vi "UDP Data Link - RTMs - Add Channels Updated.vi"(8 "error in (no error)":errorcluster, 11 "Node Ptr":u64 format="%.0x") -> (0 "error out":errorcluster)   [LabVIEW 2012, in "UDP Data Link System Explorer.lvlib"]
uses:
  UDP Data Link System Explorer.lvlib
  <vilib>/NI Veristand/Custom Device API/Custom Device Item Ref.ctl
  <vilib>/NI Veristand/Custom Device API/Custom Device Channel Type.ctl
  Shared/UDP Data Link Global.vi
  <vilib>/NI Veristand/Custom Device API/Get Item Property (String Array).vi
  <vilib>/NI Veristand/Custom Device API/Set Item Property (String Array).vi
  <vilib>/NI Veristand/Custom Device API/Custom Device API.lvlib
  <vilib>/NI Veristand/Custom Device Tools/Custom Device Utility Library/Custom Device Utility Library.lvlib
  Shared/UDP Data Link Shared.lvlib
panel:
  in  "Remove":bool
  in  "Selected Channels":i32[](listbox)
  in  "Add":bool
  in  "Available Channels":string[](tree)
  in  "OK":bool
  in  "Cancel":bool
  in  "Initial Selection":T1[](array[typedef]) format="%.0x"
  in  "Tag":string
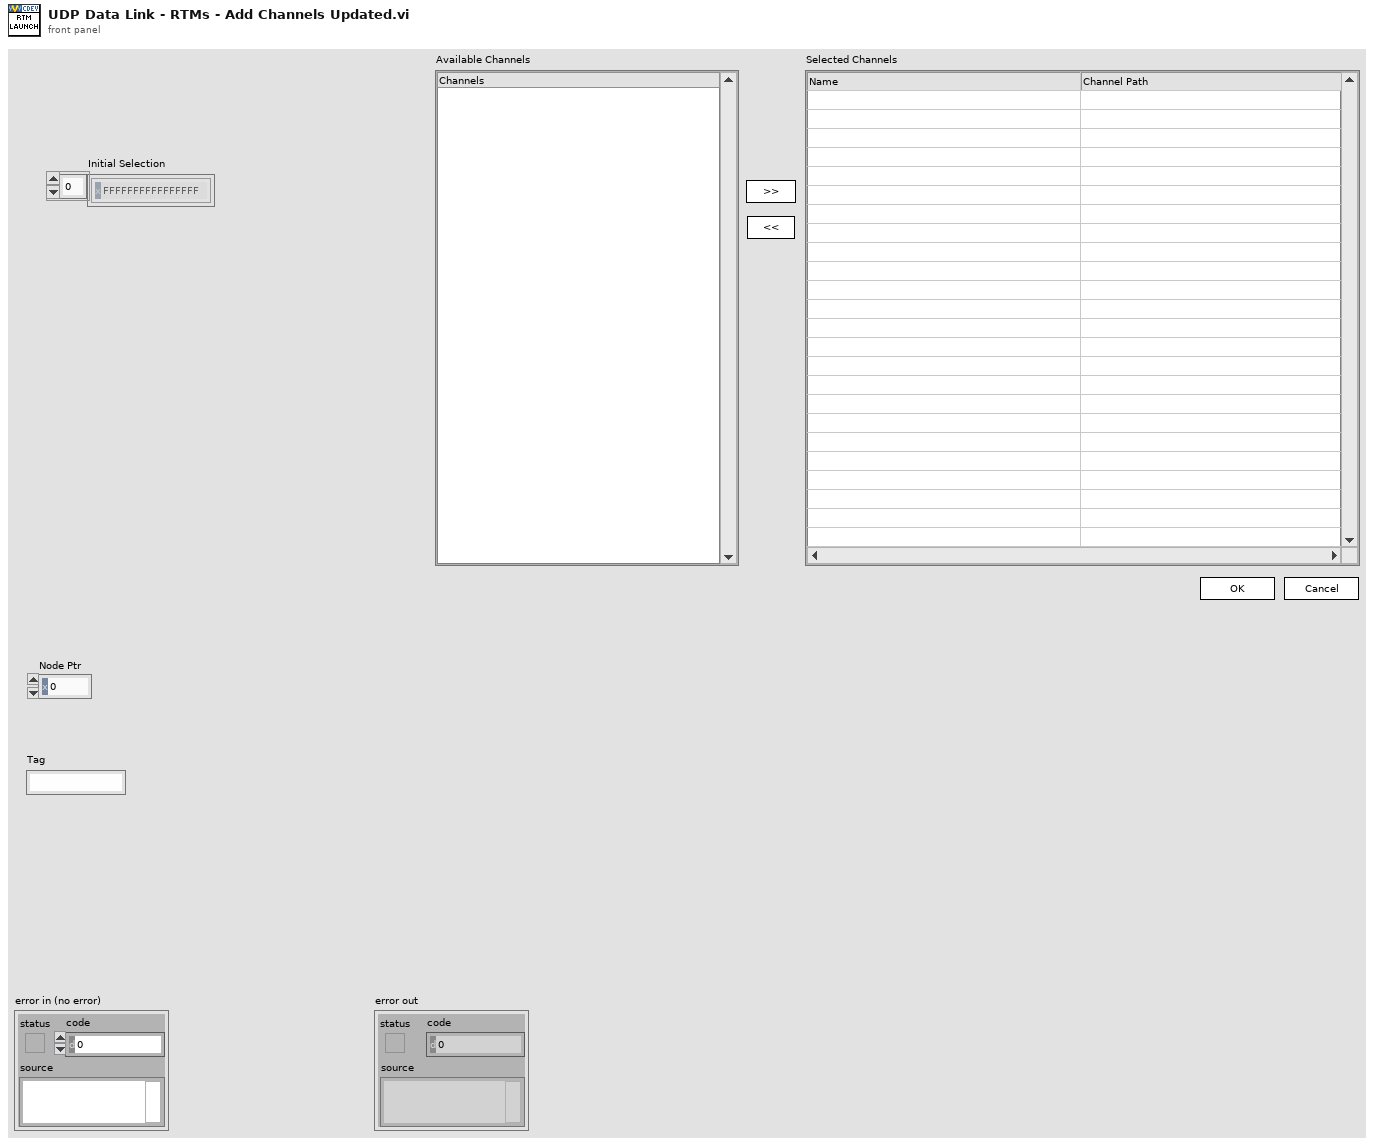
[diagram p1: front panel]
types:
  T1 = typedef "Custom Device API.lvlib/Custom Device Item Ref.ctl" = u64
  T2 = cluster{"Allow Section Selection (F)":bool, "Allow Multiple Selection (F)":bool}
  T3 = cluster{"Available Channels Label":string, "Selected Channels Label":string, "Mode":enum16{"Tx", "Rx"}}
  T4 = enum8{"Enabled", "Disabled", "Disabled and Grayed Out"}
  T5 = typedef "Custom Device API.lvlib/Custom Device Channel Type.ctl" = enum16{"Input", "Output"}
  T6 = cluster{"Tx Channel Refs":string, "Tx Channel Paths":string, "Tx Channel Names":string, "Item Ref out":T1}
  T7 = typedef "LVRowAndColumnUnsignedTypeDef.ctl" = cluster{"Row":u32, "Column":u32}
  T8 = typedef "Custom Device API.lvlib/Custom Device Item Info.ctl" = cluster{"Name":string, "Is Channel":bool, "GUID":string, "Is Waveform":bool}
  T9 = typedef "Custom Device API.lvlib/Custom Device Channel.ctl" = cluster{"Type":T5, "Units":string, "Default Value":dbl, "Faultable":bool, "Scalable":bool}
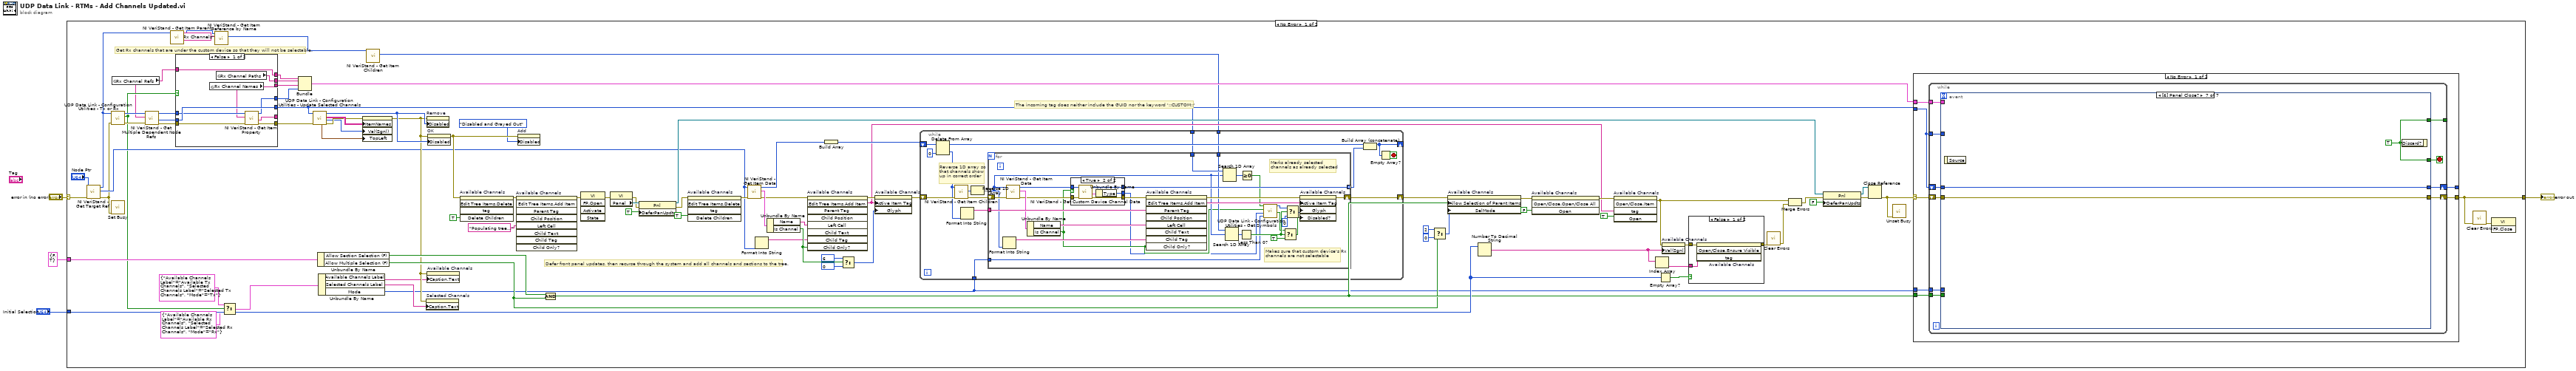
[diagram p0: block diagram]
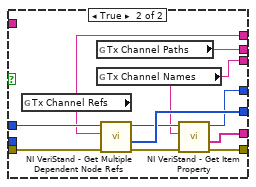
[diagram p2: hidden frame]
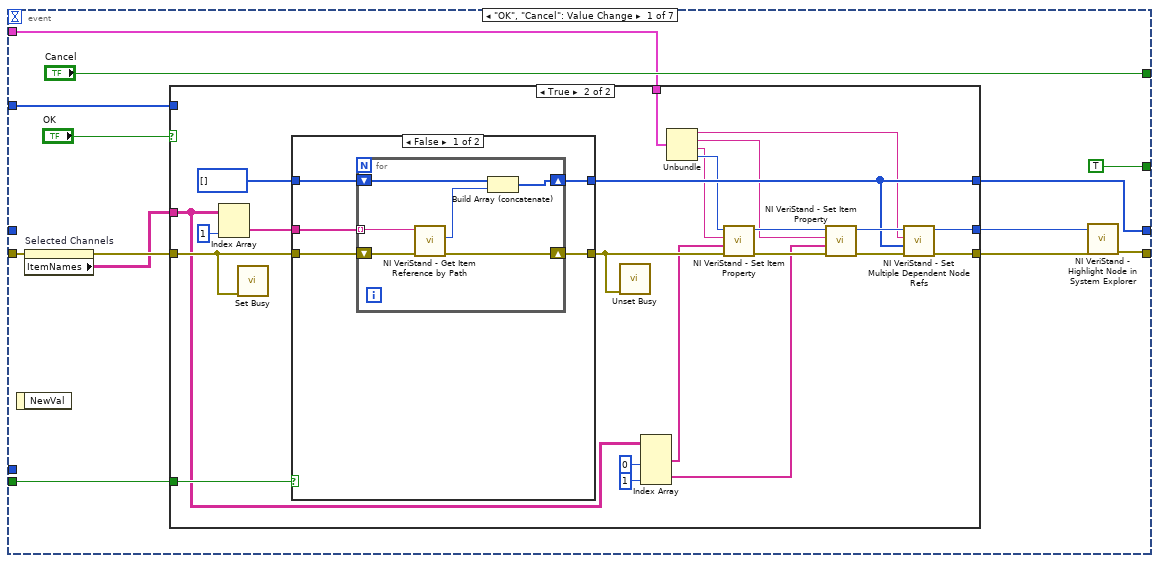
[diagram p4: hidden frame]
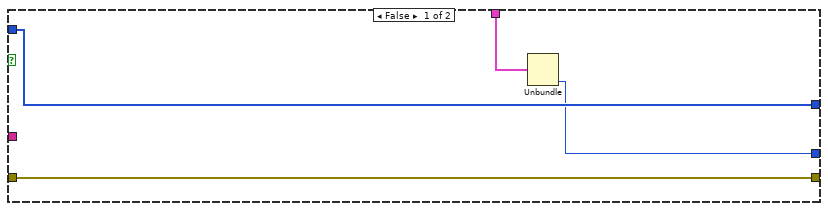
[diagram p5: hidden frame]
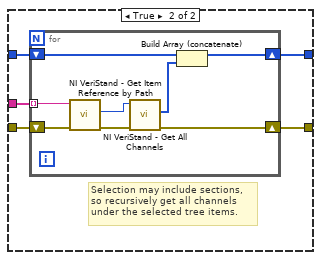
[diagram p6: hidden frame]
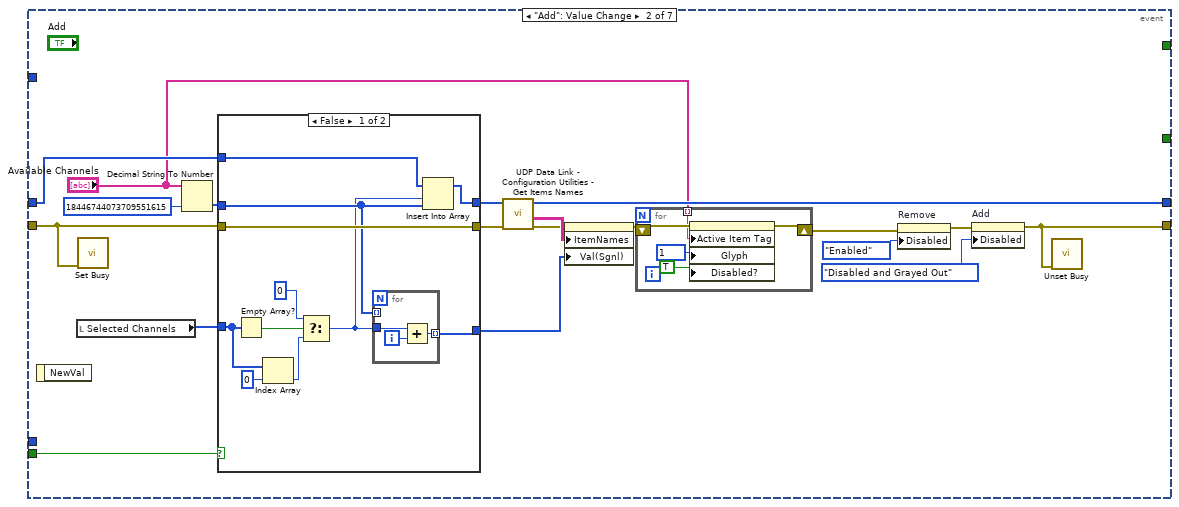
[diagram p7: hidden frame]
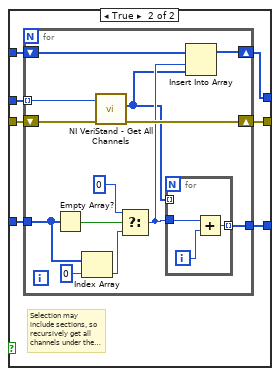
[diagram p8: hidden frame]
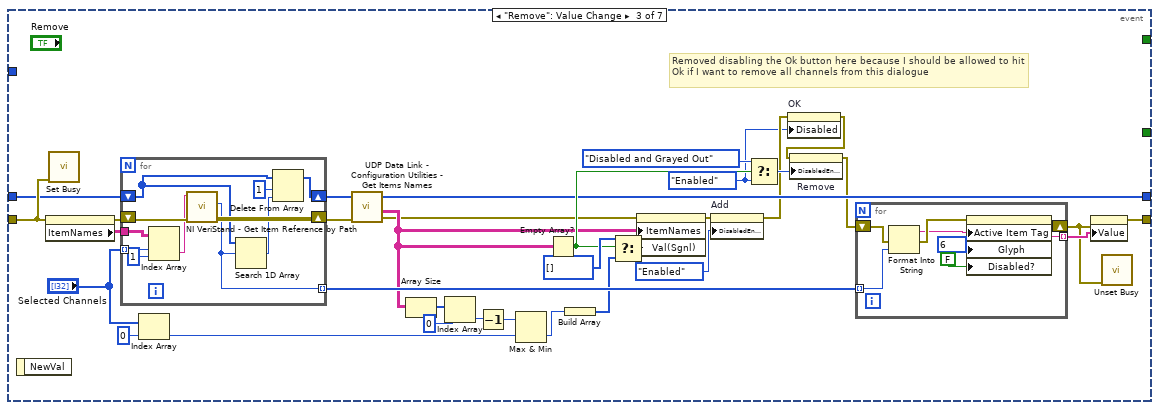
[diagram p9: hidden frame]
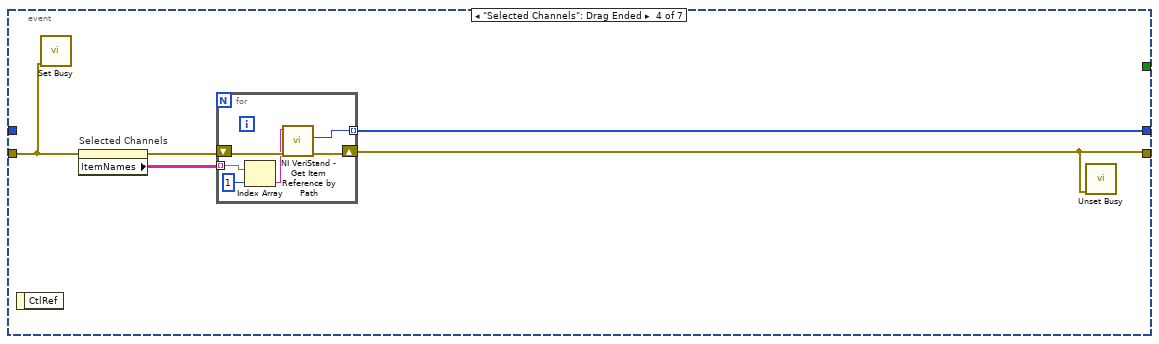
[diagram p10: hidden frame]
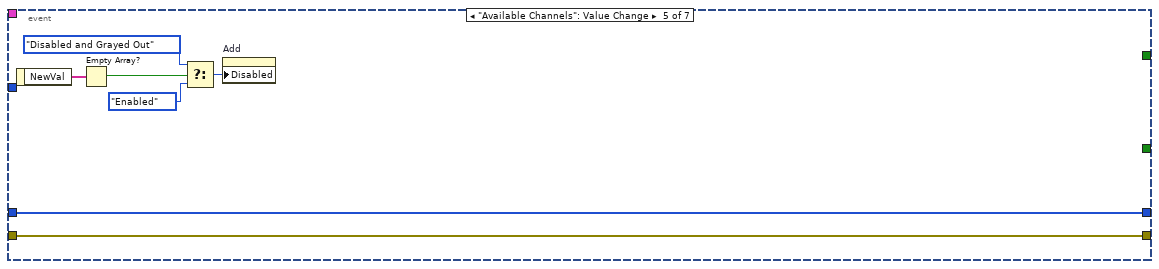
[diagram p11: hidden frame]
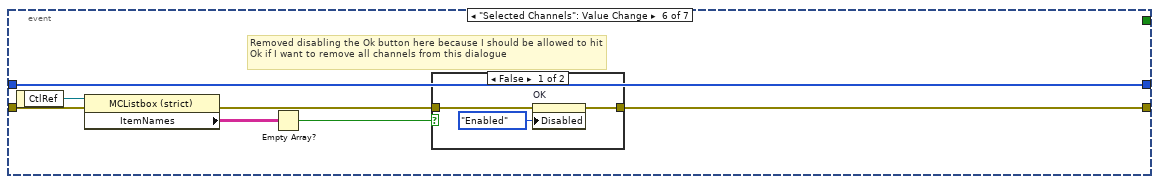
[diagram p12: hidden frame]
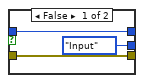
[diagram p15: hidden frame]
diagram:
  # "The incoming tag does neither include the GUID nor the keyword '::CUSTOM::'"
  n1 = case shown="No Error" "error in (no error)" {
    selector: "error in (no error)" -> [w27 w397]
    tunnel: "Initial Selection" -> [w59 _]
    tunnel: [w77 w397] -> w1
    tunnel: T2 {"Allow Section Selection (F)"=FALSE, "Allow Multiple Selection (F)"=TRUE} ("Cluster") -> [w44 _]
    frame No Error {
      # "Get Rx channels that are under the custom device so that they will not be selectable."
      # "Defer front panel updates, then recurse through the system and add all channels and sections to the tree."
      n2 = call <vilib>:"NI VeriStand - Get Target Ref.vi"("error in"=w27, "Item Ref in"="Node Ptr") -> ("error out"=w24:errorcluster, "Target Ref"=w25:T1, "Item Ref out"=w8:T1)  [unwired: 6 in, 1 out]
      n3 = call <vilib>:"Set Busy.vi"("error in (no error)"=w24) -> ()  [unwired: 3 in, 8 out]
      n4 = call "UDP Data Link - Configuration Utilities - Tx or Rx.vi"("error in (no error)"=w24, "Item Ref in"=w8) -> ("error out"=w23:errorcluster, "Tx?"=w19:bool, "Item Ref out"=w22:T1)  [unwired: 7 in]
      n5 = global read "UDP Data Link Global.vi" "Rx Channel Refs"() -> (w13:string)
      n6 = call <vilib>:"NI VeriStand - Get Multiple Dependent Node Refs.vi"("error in (no error)"=w23, "Base Property Name"=w13, "Item Ref in"=w22) -> ("error out"=w28:errorcluster, "Dependent Node Refs"=w11:T1[], "Item Ref out"=w29:T1)  [unwired: 6 in]
      n7 = call <vilib>:"NI VeriStand - Get Item Parent.vi"("Item Ref in"=w8) -> ("Parent Ref"=w6:T1)  [unwired: 7 in, 3 out]
      n8 = case shown="False" w19 {
        tunnel: w29 -> [w99 w113]
        tunnel: [w100 w112] -> w31
        tunnel: w28 -> [w96 w111]
        tunnel: [w95 w108] -> w30
        tunnel: [w94 w107] -> _
        tunnel: w11 -> [w100 _]
        tunnel: [w102 w106] -> w17
        tunnel: [w97 w105] -> w16
        tunnel: [w98 w104] -> w10
        tunnel: [w101 w103] -> w14
        tunnel: w13 -> [w101 _]
        frame False {
          n9 = global read "UDP Data Link Global.vi" "Rx Channel Names"() -> (w97:string)
          n10 = global read "UDP Data Link Global.vi" "Rx Channel Paths"() -> (w102:string)
          n11 = call-poly <vilib>:"NI VeriStand - Get Item Property.vi"("error in (no error)"=w96, "Property Name"=w97, "Item Ref in"=w99) -> ("error out"=w95:errorcluster, "Value"=w94:string[], "Item Ref out"=w98:T1)  [unwired: 1 in, 5 out]
        }
        frame True {
          n12 = global read "UDP Data Link Global.vi" "Tx Channel Refs"() -> (w103:string)
          n13 = global read "UDP Data Link Global.vi" "Tx Channel Paths"() -> (w106:string)
          n14 = global read "UDP Data Link Global.vi" "Tx Channel Names"() -> (w105:string)
          n15 = call <vilib>:"NI VeriStand - Get Multiple Dependent Node Refs.vi"("error in (no error)"=w111, "Base Property Name"=w103, "Item Ref in"=w113) -> ("error out"=w109:errorcluster, "Dependent Node Refs"=w112:T1[], "Item Ref out"=w110:T1)  [unwired: 6 in]
          n16 = call-poly <vilib>:"NI VeriStand - Get Item Property.vi"("error in (no error)"=w109, "Property Name"=w105, "Item Ref in"=w110) -> ("error out"=w108:errorcluster, "Value"=w107:string[], "Item Ref out"=w104:T1)  [unwired: 1 in, 5 out]
        }
      }
      n17 = call <vilib>:"NI VeriStand - Get Item Reference by Name.vi"("Item Name"="Rx Channels", "Parent Ref in"=w6) -> ("Item Ref"=w5:T1)  [unwired: 6 in, 3 out]
      n18 = Select(t=T3 {"Available Channels Label"="Available Tx Channels", "Selected Channels Label"="Selected Tx Channels", "Mode"=enum."Tx"} ("Parameter"), s=w19, f=T3 {"Available Channels Label"="Available Rx Channels", "Selected Channels Label"="Selected Rx Channels", "Mode"=enum."Rx"} ("Parameter")) -> (s? t:f=w18:T3)
      n19 = Bundle("Tx Channel Refs"=w14, "Tx Channel Paths"=w17, "Tx Channel Names"=w16, "Item Ref out"=w10) -> (w15:T6)  [unwired: 1 in]
      n20 = call "UDP Data Link - Configuration Utilities - Update Selected Channels.vi"("error in (no error)"=w30, "Dependent Node Refs"=w31) -> ("error out"=w40:errorcluster, "Val(Sgnl)"=w36:i32[], "Selected Channels"=w41:string[][], "Disabled Behavior"=w37:u8, "Top Left Visible Cell"=w12:T7)  [unwired: 5 in]
      n21 = Unbundle By Name(w44) -> ("Allow Section Selection (F)"=w43:bool, "Allow Multiple Selection (F)"=w42:bool)
      n22 = Unbundle By Name(w18) -> ("Available Channels Label"=w34:string, "Selected Channels Label"=w33:string, "Mode"=w32:enum16{"Tx", "Rx"})
      n23 = property on="Selected Channels" class="MCListbox (strict)"(error in=w40, "ItemNames"=w41, "Val(Sgnl)"=w36, "TopLeft"=w12) -> (error out=w35:errorcluster)  [unwired: 1 in, 1 out]
      n24 = call <vilib>:"NI VeriStand - Get Item Children.vi"("Item Ref in"=w5) -> ("Child Refs"=w9:T1[])  [unwired: 7 in, 3 out]
      n25 = property on="Selected Channels" class="MCListbox (strict)"(error in=w35, "Caption.Text"=w33) -> ()  [unwired: 1 in, 2 out]
      n26 = property on="Remove" class="Bool"(error in=w35, "Disabled"=w37) -> ()  [unwired: 1 in, 2 out]
      n27 = property on="Available Channels" class="Tree (strict)"(error in=w35, "Caption.Text"=w34) -> ()  [unwired: 1 in, 2 out]
      n28 = property on="OK" class="Bool"(error in=w35, "Disabled"=w37) -> (error out=w39:errorcluster)  [unwired: 1 in, 1 out]
      n29 = invoke on="Available Channels" class="Tree (strict)" method="Edit Tree Items.Delete"(error in=w39, "Delete Children"=TRUE ("Delete Children?")) -> (error out=w93:errorcluster)  [unwired: 3 in, 4 out]
      n30 = invoke on="Available Channels" class="Tree (strict)" method="Edit Tree Items.Add Item"(error in=w93, "Left Cell"="Populating tree..." ("Tag")) -> (error out=w90:errorcluster)  [unwired: 7 in, 8 out]
      n31 = property on="Add" class="Bool"(error in=w39, "Disabled"=T4."Disabled and Grayed Out") -> ()  [unwired: 1 in, 2 out]
      n32 = Compound Arithmetic op=AND(w43, w42) -> (w46:bool)
      n33 = invoke class="VI" method="FP.Open"(error in=w90) -> (error out=w88:errorcluster)  [unwired: 4 in, 4 out]
      n34 = property class="VI"(error in=w88) -> (error out=w86:errorcluster, "Panel"=w87:refnum<vi>)  [unwired: 1 in, 1 out]
      n35 = property class="Pnl"(reference=w87, error in=w86, "DeferPanUpdts"=TRUE ("Defer Panel Updates")) -> (reference out=w80:refnum<vi>, error out=w84:errorcluster)
      n36 = invoke on="Available Channels" class="Tree (strict)" method="Edit Tree Items.Delete"(error in=w84, "Delete Children"=TRUE ("Delete Children?")) -> (error out=w64:errorcluster)  [unwired: 3 in, 4 out]
      n37 = call <vilib>:"NI VeriStand - Get Item Data.vi"("error in (no error)"=w64, "Item Ref in"=w25) -> ("error out"=w67:errorcluster, "Item Info"=w69:T8, "Item Ref out"=w65:T1)  [unwired: 7 out]
      n38 = Format Into String(w25) -> (resulting string=w68:string)  [unwired: 3 in, 1 out]
      n39 = Unbundle By Name(w69) -> ("Name"=w70:string, "Is Channel"=w74:bool)
      n40 = invoke on="Available Channels" class="Tree (strict)" method="Edit Tree Items.Add Item"(error in=w67, "Left Cell"=w70, "Child Tag"=w68, "Child Only?"=w74) -> (error out=w71:errorcluster, "Edit Tree Items:Add Item"=w50:string)  [unwired: 5 in, 7 out]
      n41 = Build Array(w65) -> (w83:T1[])
      n42 = Select(t=6, s=w74, f=0) -> (s? t:f=w75:i32)
      n43 = property on="Available Channels" class="Tree (strict)"(error in=w71, "Active Item Tag"=w50, "Glyph"=w75) -> (error out=w66:errorcluster)  [unwired: 1 in, 1 out]
      n44 = while {
        shift-right: [w350] -> w82
        shift-left: w66 -> [w356]
        shift-right: [w355] -> _
        shift-left: w83 -> [w359]
        tunnel: w31 -> [w347]
        tunnel: w32 -> [w346]
        tunnel: w9 -> [w345]
        stop <- w354 stop-if-true
        # "Reverse 1D array so that channels show up in correct order"
        n45 = Delete From Array(array=w359, index=0) -> (deleted portion=w349:T1, array with subset deleted=w357:T1[])  [unwired: 1 in]
        n46 = call <vilib>:"NI VeriStand - Get Item Children.vi"("error in (no error)"=w356, "Item Ref in"=w349) -> ("error out"=w353:errorcluster, "Child Refs"=w352:T1[])  [unwired: 8 out]
        n47 = Format Into String(w349) -> (resulting string=w348:string)  [unwired: 3 in, 1 out]
        n48 = Reverse 1D Array(array=w352) -> (reversed array=w344:T1[])
        n49 = for {
          shift-right: [w381] -> w350
          shift-left: w353 -> [w386]
          tunnel: w344 -> [w373] mode=indexing
          tunnel: [w378] -> w351 mode=indexing
          tunnel: w348 -> [w387]
          tunnel: w347 -> [w380]
          tunnel: w346 -> [w362]
          tunnel: w345 -> [w374]
          # "Marks already selected channels as already selected"
          # "Makes sure that custom device's Rx channels are not selectable"
          n50 = Format Into String(w373) -> (resulting string=w385:string)  [unwired: 3 in, 1 out]
          n51 = call <vilib>:"NI VeriStand - Get Item Data.vi"("error in (no error)"=w386, "Item Ref in"=w373) -> ("error out"=w377:errorcluster, "Item Info"=w384:T8, "Item Ref out"=w379:T1)  [unwired: 7 out]
          n52 = Unbundle By Name(w384) -> ("Name"=w375:string, "Is Channel"=w364:bool)
          n53 = case shown="True" w364 {
            tunnel: w379 -> [w390 w396]
            tunnel: [w390 w395] -> w378
            tunnel: w377 -> [w389 w394]
            tunnel: [w389 w393] -> w376
            tunnel: [Custom_Device_Channel_Type."Input" ("Type") w391] -> w363
            frame False {
            }
            frame True {
              n54 = call <vilib>:"NI VeriStand - Get Custom Device Channel Data.vi"("error in (no error)"=w394, "Channel Ref in"=w396) -> ("error out"=w393:errorcluster, "Channel"=w392:T9, "Channel Ref out"=w395:T1)  [unwired: 4 in, 3 out]
              n55 = Unbundle By Name(w392) -> ("Type"=w391:T5)
            }
          }
          n56 = invoke on="Available Channels" class="Tree (strict)" method="Edit Tree Items.Add Item"(error in=w376, "Parent Tag"=w387, "Left Cell"=w375, "Child Tag"=w385, "Child Only?"=w364) -> (error out=w383:errorcluster, "Edit Tree Items:Add Item"=w382:string)  [unwired: 4 in, 7 out]
          n57 = Search 1D Array(1D array=w380, element=w373) -> (index of element=w366:i32)  [unwired: 1 in]
          n58 = Search 1D Array(1D array=w374, element=w373) -> (index of element=w372:i32)  [unwired: 1 in]
          n59 = Less Than 0?(x=w372) -> (x < 0?=w368:bool)
          n60 = Greater Or Equal To 0?(x=w366) -> (x >= 0?=w365:bool)
          n61 = call "UDP Data Link - Configuration Utilities - Get Symbols.vi"("Mode"=w362, "Channel Type"=w363, "Is Channel?"=w364, "Is Selected?"=w365) -> ("Disabled?"=w360:bool, "Symbole"=w361:i32)  [unwired: 6 in]
          n62 = Select(t=w360, s=w368, f=TRUE) -> (s? t:f=w371:bool)
          n63 = Select(t=w361, s=w368, f=0) -> (s? t:f=w369:i32)
          n64 = property on="Available Channels" class="Tree (strict)"(error in=w383, "Active Item Tag"=w382, "Glyph"=w369, "Disabled?"=w371) -> (error out=w381:errorcluster)  [unwired: 1 in, 1 out]
        }
        n65 = Build Array (concatenate)(w357, w351) -> (w355:T1[])
        n66 = Empty Array?(array=w355) -> (empty?=w354:bool)
      }
      n67 = Select(t=2 ("Selection Mode"), s=w42, f=0 ("Selection Mode")) -> (s? t:f=w47:i32)
      n68 = property on="Available Channels" class="Tree (strict)"(error in=w82, "Allow Selection of Parent Items"=w46, "SelMode"=w47) -> (error out=w55:errorcluster)  [unwired: 1 in, 1 out]
      n69 = Number To Decimal String(number=w59) -> (decimal integer string=w57:string[])  [unwired: 1 out]
      n70 = invoke on="Available Channels" class="Tree (strict)" method="Open/Close.Open/Close All"(error in=w55, "Open"=FALSE ("Open?")) -> (error out=w53:errorcluster)  [unwired: 2 in, 3 out]
      n71 = invoke on="Available Channels" class="Tree (strict)" method="Open/Close.Item"(error in=w53, "tag"=w50, "Open"=TRUE ("Open?")) -> (error out=w51:errorcluster)  [unwired: 2 in, 4 out]
      n72 = Index Array(array=w57) -> (element=w56:string)  [unwired: 1 in]
      n73 = Empty Array?(array=w59) -> (empty?=w58:bool)
      n74 = property on="Available Channels" class="Tree (strict)"(error in=w51, "Val(Sgnl)"=w57) -> (error out=w61:errorcluster)  [unwired: 1 in, 1 out]
      n75 = case shown="False" w58 {
        tunnel: w61 -> [w116 w117]
        tunnel: [w115 w117] -> w60
        tunnel: w56 -> [w114 _]
        frame False {
          n76 = invoke on="Available Channels" class="Tree (strict)" method="Open/Close.Ensure Visible"(error in=w116, "tag"=w114) -> (error out=w115:errorcluster)  [unwired: 2 in, 3 out]
        }
        frame True {
        }
      }
      n77 = call <vilib>:"Clear Errors.vi"("error in (no error)"=w60) -> ("error out"=w63:errorcluster)  [unwired: 6 out]
      n78 = Merge Errors(w51, w63) -> (w62:errorcluster)
      n79 = property class="Pnl"(reference=w80, error in=w62, "DeferPanUpdts"=FALSE ("Defer Panel Updates")) -> (reference out=w78:refnum<vi>, error out=w79:errorcluster)
      n80 = Close Reference(reference=w78, error in (no error)=w79) -> (error out=w45:errorcluster)
      n81 = call <vilib>:"Unset Busy.vi"("error in (no error)"=w45) -> ()  [unwired: 1 in, 10 out]
      n82 = case shown="No Error" w45 {
        selector: w45 -> [w124 w343]
        tunnel: [w123 w343] -> w77
        tunnel: [w122 w342] -> _
        tunnel: w46 -> [w121 _]
        tunnel: w31 -> [w120 w342]
        tunnel: w32 -> [w119 _]
        tunnel: w15 -> [w118 _]
        frame No Error {
          n83 = while {
            shift-right: [w133] -> w123
            shift-left: w124 -> [w134]
            tunnel: [w132] -> _
            tunnel: w121 -> [w130]
            shift-right: [w127] -> w122
            shift-left: w120 -> [w129]
            tunnel: w120 -> [w128]
            tunnel: w119 -> [w126]
            tunnel: w118 -> [w125]
            stop <- w131 stop-if-true
            n84 = event shown="[6] Panel Close?" {
              selector: _ -> [_ _ _ _ _ _ _]
              dyn-events: _ -> [_ _ _ _ _ _ _]
              timeout: _ -> [_ _ _ _ _ _ _]
              tunnel: w134 -> [w143 w215 w291 w314 w327 w332 w341]
              tunnel: [w139 w199 w264 w311 w327 w329 w341] -> w133
              tunnel: ["Cancel" _ _ _ _ _ w340] -> w132
              tunnel: [TRUE ("Discard?") _ _ _ _ _ w340] -> w131
              tunnel: [w135 w211 w270 w310 w324 w334 w339] -> w127
              tunnel: w130 -> [w145 w214 _ _ _ _ _]
              tunnel: w129 -> [_ w213 w288 _ w324 w334 w339]
              tunnel: w128 -> [w141 _ _ _ _ _ _]
              tunnel: w126 -> [_ _ _ _ _ _ _]
              tunnel: w125 -> [w138 _ _ _ _ _ _]
              event "OK", "Cancel": Value Change {
                n85 = event-data() -> ()  [unwired: 2 out]
                n86 = property on="Selected Channels" class="MCListbox (strict)"(error in=w143) -> (error out=w142:errorcluster, "ItemNames"=w140:string[][])  [unwired: 1 in, 1 out]
                n87 = case shown="True" "OK" {
                  tunnel: w140 -> [_ w163]
                  tunnel: w145 -> [_ w174]
                  tunnel: w142 -> [w151 w172]
                  tunnel: [w150 w159] -> w135
                  tunnel: [w151 w161] -> w136
                  tunnel: w141 -> [w150 _]
                  tunnel: w138 -> [w149 w160]
                  tunnel: [w148 w152] -> w137
                  frame False {
                    n88 = Unbundle(w149) -> ("Item Ref out"=w148:T1)  [unwired: 3 out]
                  }
                  frame True {
                    n89 = Index Array(array=w163, index (col)=1 ("disabled index (col)")) -> (element=w170:string[])  [unwired: 1 in]
                    n90 = call <vilib>:"Set Busy.vi"("error in (no error)"=w172) -> ()  [unwired: 3 in, 8 out]
                    n91 = case shown="False" w174 {
                      tunnel: w172 -> [w179 w190]
                      tunnel: [w175 w188] -> w159
                      tunnel: [w178 w187] -> w162
                      tunnel: T1[] [] ("Channel Refs") -> [w176 w189]
                      tunnel: w170 -> [w177 w186]
                      frame False {
                        n92 = for {
                          tunnel: w177 -> [w183] mode=indexing
                          shift-right: [w180] -> w175
                          shift-left: w176 -> [w181]
                          shift-right: [w184] -> w178
                          shift-left: w179 -> [w185]
                          n93 = call <vilib>:"NI VeriStand - Get Item Reference by Path.vi"("error in (no error)"=w185, "Item Path in"=w183) -> ("error out"=w184:errorcluster, "Item Ref"=w182:T1)  [unwired: 6 in, 2 out]
                          n94 = Build Array (concatenate)(w181, w182) -> (w180:T1[])
                        }
                      }
                      frame True {
                        # "Selection may include sections, so recursively get all channels under the selected tree items."
                        n95 = for {
                          shift-right: [w196] -> w188
                          shift-left: w189 -> [w197]
                          shift-right: [w198] -> w187
                          shift-left: w190 -> [w193]
                          tunnel: w186 -> [w194] mode=indexing
                          n96 = call <vilib>:"NI VeriStand - Get Item Reference by Path.vi"("error in (no error)"=w193, "Item Path in"=w194) -> ("error out"=w192:errorcluster, "Item Ref"=w191:T1)  [unwired: 6 in, 2 out]
                          n97 = call <vilib>:"NI VeriStand - Get All Channels.vi"("error in"=w192, "Section Ref in"=w191) -> ("error out"=w198:errorcluster, "Channel Refs"=w195:T1[])  [unwired: 8 out]
                          n98 = Build Array (concatenate)(w197, w195) -> (w196:T1[])
                        }
                      }
                    }
                    n99 = call <vilib>:"Unset Busy.vi"("error in (no error)"=w162) -> ()  [unwired: 1 in, 10 out]
                    n100 = Index Array(array=w163, index (col) #1=0 ("disabled index (col)"), index (col) #2=1 ("index (col)")) -> (element #1=w156:string[], element #2=w154:string[])  [unwired: 2 in]
                    n101 = Unbundle(w160) -> ("Tx Channel Refs"=w153:string, "Tx Channel Paths"=w155:string, "Tx Channel Names"=w157:string, "Item Ref out"=w158:T1)
                    n102 = call-poly <vilib>:"NI VeriStand - Set Item Property.vi"("error in (no error)"=w162, "Value"=w156, "Property Name"=w157, "Item Ref in"=w158) -> ("error out"=w164:errorcluster, "Item Ref out"=w165:T1)  [unwired: 5 in, 1 out]
                    n103 = call-poly <vilib>:"NI VeriStand - Set Item Property.vi"("error in (no error)"=w164, "Value"=w154, "Property Name"=w155, "Item Ref in"=w165) -> ("error out"=w168:errorcluster, "Item Ref out"=w169:T1)  [unwired: 5 in, 1 out]
                    n104 = call <vilib>:"NI VeriStand - Set Multiple Dependent Node Refs.vi"("error in (no error)"=w168, "Dependent Node Refs"=w159, "Base Property Name"=w153, "Item Ref in"=w169) -> ("error out"=w161:errorcluster, "Item Ref out"=w152:T1)  [unwired: 6 in]
                  }
                }
                n105 = call <vilib>:"NI VeriStand - Highlight Node in System Explorer.vi"("error in (no error)"=w136, "Item Ref in"=w137) -> ("error out"=w139:errorcluster)  [unwired: 8 in, 1 out]
              }
              event "Add": Value Change {
                n106 = event-data() -> ()  [unwired: 2 out]
                n107 = local read "Selected Channels"() -> (w203:i32[])
                n108 = call <vilib>:"Set Busy.vi"("error in (no error)"=w215) -> ()  [unwired: 3 in, 8 out]
                n109 = Decimal String To Number(string="Available Channels", default (0L)=T1 18446744073709551615 ("Device Item Ref")) -> (number=w217:u64[])  [unwired: 2 out]
                n110 = case shown="False" w214 {
                  tunnel: w215 -> [w233 w243]
                  tunnel: [w230 w242] -> w212
                  tunnel: w217 -> [w225 w241]
                  tunnel: [w233 w240] -> w210
                  tunnel: w213 -> [w231 w239]
                  tunnel: w203 -> [w229 w238]
                  tunnel: [w223 w237] -> w202
                  frame False {
                    n111 = Empty Array?(array=w229) -> (empty?=w232:bool)
                    n112 = Index Array(array=w229, index=0) -> (element=w227:i32)
                    n113 = Select(t=0, s=w232, f=w227) -> (s? t:f=w224:i32)
                    n114 = for {
                      tunnel: w225 -> [_] mode=indexing
                      tunnel: w224 -> [w236]
                      tunnel: [w234] -> w223 mode=indexing
                      i -> [w235]
                      n115 = Add(x=w236, y=w235) -> (x+y=w234:i32)
                    }
                    n116 = Insert Into Array(array=w231, index=w224, new element=w225) -> (w230:T1[])
                  }
                  frame True {
                    # "Selection may include sections, so recursively get all channels under the selected tree items."
                    n117 = for {
                      shift-right: [w248] -> w242
                      shift-left: w239 -> [w247]
                      shift-right: [w255] -> w240
                      shift-left: w243 -> [w256]
                      tunnel: w241 -> [w254] mode=indexing
                      tunnel: w238 -> [w249]
                      tunnel: [w246] -> w237
                      n118 = Empty Array?(array=w249) -> (empty?=w250:bool)
                      n119 = Index Array(array=w249, index=0) -> (element=w252:i32)
                      n120 = call <vilib>:"NI VeriStand - Get All Channels.vi"("error in"=w256, "Section Ref in"=w254) -> ("error out"=w255:errorcluster, "Channel Refs"=w244:T1[])  [unwired: 8 out]
                      n121 = Select(t=0, s=w250, f=w252) -> (s? t:f=w245:i32)
                      n122 = for {
                        tunnel: w245 -> [w259]
                        tunnel: [w257] -> w246 mode=indexing
                        tunnel: w244 -> [_] mode=indexing
                        i -> [w258]
                        n123 = Add(x=w259, y=w258) -> (x+y=w257:i32)
                      }
                      n124 = Insert Into Array(array=w247, index=w245, new element=w244) -> (w248:T1[])
                    }
                  }
                }
                n125 = call "UDP Data Link - Configuration Utilities - Get Items Names.vi"("error IO 2"=w210, "TCP Channel Refs In"=w212) -> ("error IO"=w205:errorcluster, "Items Names"=w206:string[][], "TCP Channel Refs Out"=w211:T1[])  [unwired: 7 in]
                n126 = property on="Selected Channels" class="MCListbox (strict)"(error in=w205, "ItemNames"=w206, "Val(Sgnl)"=w202) -> (error out=w209:errorcluster)  [unwired: 1 in, 1 out]
                n127 = for {
                  shift-right: [w221] -> w201
                  shift-left: w209 -> [w222]
                  tunnel: "Available Channels" -> [w219] mode=indexing
                  n128 = property on="Available Channels" class="Tree (strict)"(error in=w222, "Active Item Tag"=w219, "Glyph"=1, "Disabled?"=TRUE ("Active Item:Disabled?")) -> (error out=w221:errorcluster)  [unwired: 1 in, 1 out]
                }
                n129 = property on="Remove" class="Bool"(error in=w201, "Disabled"=T4."Enabled") -> (error out=w200:errorcluster)  [unwired: 1 in, 1 out]
                n130 = property on="Add" class="Bool"(error in=w200, "Disabled"=T4."Disabled and Grayed Out") -> (error out=w199:errorcluster)  [unwired: 1 in, 1 out]
                n131 = call <vilib>:"Unset Busy.vi"("error in (no error)"=w199) -> ()  [unwired: 1 in, 10 out]
              }
              event "Remove": Value Change {
                w261 = T4."Enabled" ("Disabled")
                # "Removed disabling the Ok button here because I should be allowed to hit Ok if I want to remove all channels from this dialogue"
                n132 = event-data() -> ()  [unwired: 2 out]
                n133 = property on="Selected Channels" class="MCListbox (strict)"(error in=w291) -> (error out=w290:errorcluster, "ItemNames"=w289:string[][])  [unwired: 1 in, 1 out]
                n134 = call <vilib>:"Set Busy.vi"("error in (no error)"=w291) -> ()  [unwired: 3 in, 8 out]
                n135 = for {
                  tunnel: w289 -> [w300]
                  tunnel: "Selected Channels" -> [w301] mode=indexing
                  shift-right: [w299] -> w272
                  shift-left: w290 -> [w302]
                  shift-right: [w297] -> w269
                  shift-left: w288 -> [w298]
                  tunnel: [w294] -> w287 mode=indexing
                  n136 = Index Array(array=w300, index (row)=w301, index (col)=1 ("disabled index (col)")) -> (element=w292:string)
                  n137 = call <vilib>:"NI VeriStand - Get Item Reference by Path.vi"("error in (no error)"=w302, "Item Path in"=w292) -> ("error out"=w299:errorcluster, "Item Ref"=w294:T1)  [unwired: 6 in, 2 out]
                  n138 = Search 1D Array(1D array=w298, element=w294) -> (index of element=w295:i32)  [unwired: 1 in]
                  n139 = Delete From Array(array=w298, length=1, index=w295) -> (array with subset deleted=w297:T1[])  [unwired: 1 out]
                }
                n140 = Index Array(array="Selected Channels", index=0) -> (element=w275:i32)
                n141 = call "UDP Data Link - Configuration Utilities - Get Items Names.vi"("error IO 2"=w272, "TCP Channel Refs In"=w269) -> ("error IO"=w268:errorcluster, "Items Names"=w271:string[][], "TCP Channel Refs Out"=w270:T1[])  [unwired: 7 in]
                n142 = Array Size(array=w271) -> (size(s)=w279:i32[])
                n143 = Index Array(array=w279, index=0) -> (element=w277:i32)
                n144 = Decrement(x=w277) -> (x-1=w276:i32)
                n145 = Max & Min(x=w276, y=w275) -> (min(x,y)=w274:i32)  [unwired: 1 out]
                n146 = Empty Array?(array=w271) -> (empty?=w284:bool)
                n147 = Build Array(w274) -> (w281:i32[])
                n148 = Select(t=i32[] [] ("Selected TCP Channels"), s=w284, f=w281) -> (s? t:f=w285:i32[])
                n149 = property on="Selected Channels" class="MCListbox (strict)"(error in=w268, "ItemNames"=w271, "Val(Sgnl)"=w285) -> ()  [unwired: 1 in, 2 out]
                n150 = property on="Add" class="Bool"(error in=w268, "DisabledEnum"=T4."Enabled" ("Disabled")) -> (error out=w267:errorcluster)  [unwired: 1 in, 1 out]
                n151 = Select(t=T4."Disabled and Grayed Out" ("Disabled"), s=w284, f=w261) -> (s? t:f=w283:T4)
                n152 = property on="OK" class="Bool"(error in=w267, "Disabled"=w261) -> (error out=w266:errorcluster)  [unwired: 1 in, 1 out]
                n153 = property on="Remove" class="Bool"(error in=w266, "DisabledEnum"=w283) -> (error out=w265:errorcluster)  [unwired: 1 in, 1 out]
                n154 = for {
                  shift-right: [w307] -> w263
                  shift-left: w265 -> [w305]
                  tunnel: w287 -> [w306] mode=indexing
                  tunnel: [w303] -> w273 mode=indexing
                  n155 = Format Into String(error in=w305, w306) -> (resulting string=w303:string, error out=w304:errorcluster)  [unwired: 2 in]
                  n156 = property on="Available Channels" class="Tree (strict)"(error in=w304, "Active Item Tag"=w303, "Glyph"=6, "Disabled?"=FALSE ("Active Item:Disabled?")) -> (error out=w307:errorcluster)  [unwired: 1 in, 1 out]
                }
                n157 = property on="Available Channels" class="Tree (strict)"(error in=w263, "Value"=w273) -> (error out=w264:errorcluster)  [unwired: 1 in, 1 out]
                n158 = call <vilib>:"Unset Busy.vi"("error in (no error)"=w263) -> ()  [unwired: 1 in, 10 out]
              }
              event "Selected Channels": Drag Ended {
                n159 = event-data() -> ()  [unwired: 2 out]
                n160 = call <vilib>:"Set Busy.vi"("error in (no error)"=w314) -> ()  [unwired: 3 in, 8 out]
                n161 = property on="Selected Channels" class="MCListbox (strict)"(error in=w314) -> (error out=w313:errorcluster, "ItemNames"=w312:string[][])  [unwired: 1 in, 1 out]
                n162 = for {
                  tunnel: w312 -> [w319] mode=indexing
                  shift-right: [w318] -> w311
                  shift-left: w313 -> [w320]
                  tunnel: [w317] -> w310 mode=indexing
                  n163 = Index Array(array=w319, index=1 ("disabled index (col)")) -> (element=w316:string)
                  n164 = call <vilib>:"NI VeriStand - Get Item Reference by Path.vi"("error in (no error)"=w320, "Item Path in"=w316) -> ("error out"=w318:errorcluster, "Item Ref"=w317:T1)  [unwired: 6 in, 2 out]
                }
                n165 = call <vilib>:"Unset Busy.vi"("error in (no error)"=w311) -> ()  [unwired: 1 in, 10 out]
              }
              event "Available Channels": Value Change {
                n166 = event-data() -> ("NewVal"=w326:string[])  [unwired: 1 out]
                n167 = Empty Array?(array=w326) -> (empty?=w323:bool)
                n168 = Select(t=T4."Disabled and Grayed Out" ("Disabled"), s=w323, f=T4."Enabled" ("Disabled")) -> (s? t:f=w325:T4)
                n169 = property on="Add" class="Bool"("Disabled"=w325) -> ()  [unwired: 2 in, 2 out]
              }
              event "Selected Channels": Value Change {
                # "Removed disabling the Ok button here because I should be allowed to hit Ok if I want to remove all channels from this dialogue"
                n170 = event-data() -> ("CtlRef"=w333:refnum<vi>)  [unwired: 1 out]
                n171 = property class="MCListbox (strict)"(reference=w333, error in=w332) -> (error out=w330:errorcluster, "ItemNames"=w331:string[][])  [unwired: 1 out]
                n172 = Empty Array?(array=w331) -> (empty?=w328:bool)
                n173 = case shown="False" w328 {
                  tunnel: w330 -> [w337 w338]
                  tunnel: [w336 w338] -> w329
                  frame False {
                    n174 = property on="OK" class="Bool"(error in=w337, "Disabled"=T4."Enabled") -> (error out=w336:errorcluster)  [unwired: 1 in, 1 out]
                  }
                  frame True {
                  }
                }
              }
              event Panel Close? {
                w340 = TRUE ("Discard?")
                n175 = event-data() -> ()  [unwired: 2 out]
                n176 = event-data("Discard?"=w340) -> ()  [unwired: 1 in, 1 out]
              }
            }
          }
        }
        frame Error {
        }
      }
      n177 = call <vilib>:"Clear Errors.vi"("error in (no error)"=w77) -> ("error out"=w76:errorcluster)  [unwired: 6 out]
      n178 = invoke class="VI" method="FP.Close"(error in=w76) -> ()  [unwired: 2 in, 3 out]
    }
    frame Error {
    }
  }
  "error out" <- w1
